vi "scaninput.vi"(8 "error in (no error)":errorcluster, 11 "16InOut in":refnum<class "16InOut.lvclass">) -> (0 "error out":errorcluster, 3 "16InOut out":refnum<class "16InOut.lvclass">)   [LabVIEW 2019, in "16InOut.lvclass"]
uses:
  16InOut.lvclass
  C:/Users/user/Desktop/204J1/System/Function/IO Folder/IO_Class/IOCard.lvclass
  IOCard.lvclass/IOCard.ctl
  IOCard.lvclass
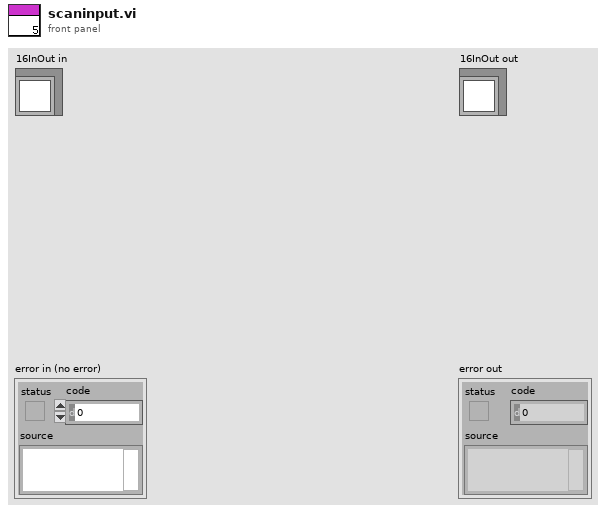
[diagram p1: front panel]
types:
  T1 = typedef "IO Card_Type.ctl" = enum16{"None", "Unidaq32", "6480", "2410C-64", "Zan", "DMC1000B", "16InOut", "Robot", "DMC3600"}
  T2 = cluster{"IO Card Type":T1, "IOType":enum16{"Input", "Output"}, "CardNumber":i32, "ConnectAct":bool, "IP":string}
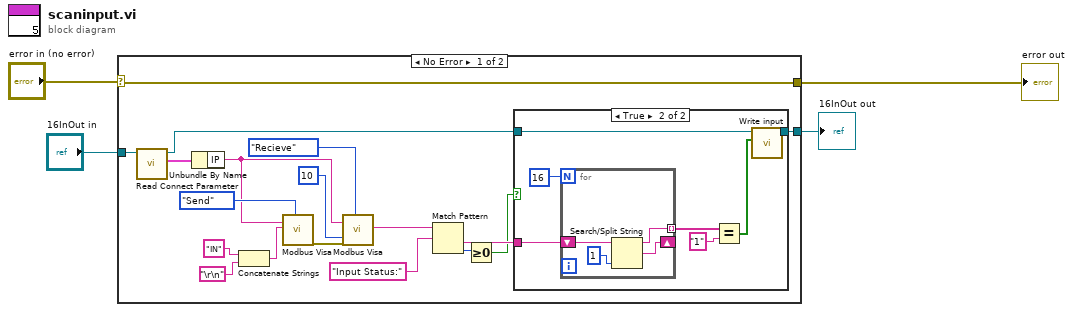
[diagram p0: block diagram]
diagram:
  n1 = case shown="No Error" "error in (no error)" {
    selector: "error in (no error)" -> [w9 w35]
    tunnel: "16InOut in" -> [w22 w36]
    tunnel: [w17 w36] -> w2
    tunnel: [w9 w35] -> w1
    frame No Error {
      n2 = call "Read Connect Parameter.vi"("IOCard in"=w22) -> ("Connect Parameter"=w20:T2, "IOCard out"=w18:refnum<class "16InOut.lvclass">)  [unwired: 8 in, 1 out]
      n3 = Unbundle By Name(w20) -> ("IP"=w15:string)
      n4 = Concatenate Strings("IN" ("Cmd"), "\r\n") -> (w8:string)
      n5 = call "Modbus Visa.vi"("VISA resource name"=w15, "Cmd"=w8, "VisaAction"=enum16{"Open", "Send", "Recieve", "Close"}."Send") -> ("error out"=w14:errorcluster)  [unwired: 15 in, 1 out]
      n6 = call "Modbus Visa.vi"("VISA resource name"=w15, "Time(0.1)"=u32 10, "error in (no error)"=w14, "VisaAction"=enum16{"Open", "Send", "Recieve", "Close"}."Recieve") -> ("read string"=w12:string)  [unwired: 14 in, 1 out]
      n7 = Match Pattern(string=w12, regular expression="Input Status:") -> (after substring=w10:string, offset past match=w6:i32)  [unwired: 1 in, 2 out]
      n8 = Greater Or Equal To 0?(x=w6) -> (x >= 0?=w5:bool)
      n9 = case shown="True" w5 {
        tunnel: w18 -> [w23 w30]
        tunnel: [w23 w29] -> w17
        tunnel: w10 -> [_ w28]
        frame False {
        }
        frame True {
          n10 = for {
            N: 16 -> [_]
            shift-right: [w32] -> _
            shift-left: w28 -> [w34]
            tunnel: [w31] -> w27 mode=indexing
            n11 = Search/Split String(string=w34, offset (0)=1) -> (substring before match=w31:string, match + rest of string=w32:string)  [unwired: 1 in, 1 out]
          }
          n12 = Equal?(x=w27, y="1") -> (x = y?=w25:bool[])
          n13 = call-dynamic "Write input.vi"("input"=w25, "IOCard in"=w30) -> ("IOCard out"=w29:refnum<class "16InOut.lvclass">)  [unwired: 8 in, 1 out]
        }
      }
    }
    frame Error {
    }
  }
  "error out" <- w1
  "16InOut out" <- w2
